vi "Const Lang Default English.vi"() -> (3 "UI Descriptions":T1={"Main Panel"={"Title"={"Frame Num"={"Name"="Frame Num", "Tip"="", "Description"=""}, "Name"={"Name"="Name", "Tip"="", "Description"=""}}, "Frame Basic"={"pic"={"Name"="pic", "Tip"="", "Description"=""}, "state"={"Name"="state", "Tip"="", "Description"=""}, "wait"={"Name"="wait", "Tip"="", "Description"=""}, "next"={"Name"="next", "Tip"="Next frame number", "Description"="Next frame number  \n999: Return to frame number 0  \n1000: Remove object  \n12XX: Invisible, where XX represents the duration  \nA minus sign indicates direction reversal"}, "dvx"={"Name"="dvx", "Tip"="movement speed", "Description"="Forward (positive) and backward (negative) movement speed"}, "dvy"={"Name"="dvy", "Tip"="movement speed", "Description"="Upward (negative) and downward (positive) movement speed"}, "dvz"={"Name"="dvz", "Tip"="movement speed", "Description"="Vertical movement speed, with the direction determined by the ◆ and □ arrow keys"}, "centerx"={"Name"="centerx", "Tip"="X-axis position of the frame center", "Description"="X-axis position of the frame center (shadow), with direction from left to right"}, "centery"={"Name"="centery", "Tip"="Y-axis position of the frame center", "Description"="Y-axis position of the frame center (shadow), with direction from top to bottom"}, "sound"={"Name"="sound", "Tip"="", "Description"=""}}, "Frame Skill"={"mp"={"Name"="mp", "Tip"="HP/MP Consumption", "Description"="HP/MP Consumption  \nOOXXX: OO represents the tens digit of HP consumption, XXX represents MP consumption  \n100: Consumes 100 MP  \n4300: Consumes 40 HP and 300 MP  \n\nWhen entering a frame using hit_XX:  \n  - Positive values indicate consumption  \n  - Negative values indicate recovery  \n\nWhen entering a frame using next:  \n  - Positive values have no effect  \n  - Negative values indicate consumption"}, "hit_a"={"Name"="hit_a", "Tip"="When pressing Attack, jump to the corresponding frame number", "Description"="When pressing Attack, jump to the corresponding frame number"}, "hit_d"={"Name"="hit_d", "Tip"="When pressing Defense, jump to the corresponding frame number", "Description"="When pressing Defense, jump to the corresponding frame number"}, "hit_j"={"Name"="hit_j", "Tip"="When pressing Jump, jump to the corresponding frame number", "Description"="When pressing Jump, jump to the corresponding frame number"}, "hit_Fa"={"Name"="hit_Fa", "Tip"="When pressing Defense △ Attack, jump to the corresponding frame number", "Description"="When pressing Defense △ Attack, jump to the corresponding frame number"}, "hit_Ua"={"Name"="hit_Ua", "Tip"="When pressing Defense ◆ Attack, jump to the corresponding frame number", "Description"="When pressing Defense ◆ Attack, jump to the corresponding frame number"}, "hit_Da"={"Name"="hit_Da", "Tip"="When pressing Defense □ Attack, jump to the corresponding frame number", "Description"="When pressing Defense □ Attack, jump to the corresponding frame number"}, "hit_Fj"={"Name"="hit_Fj", "Tip"="When pressing Defense △ Jump, jump to the corresponding frame number", "Description"="When pressing Defense △ Jump, jump to the corresponding frame number"}, "hit_Uj"={"Name"="hit_Uj", "Tip"="When pressing Defense ◆ Jump, jump to the corresponding frame number", "Description"="When pressing Defense ◆ Jump, jump to the corresponding frame number"}, "hit_Dj"={"Name"="hit_Dj", "Tip"="When pressing Defense □ Jump, jump to the corresponding frame number", "Description"="When pressing Defense □ Jump, jump to the corresponding frame number"}, "hit_ja"={"Name"="hit_ja", "Tip"="When pressing Defense + Jump + Attack, jump to the corresponding frame number", "Description"="When pressing Defense + Jump + Attack, jump to the corresponding frame number"}}, "bp"={"x"={"Name"="x", "Tip"="X-axis position of mouth bleeding", "Description"="X-axis position of mouth bleeding\nBleeding occurs when HP is less than 1/3"}, "y"={"Name"="y", "Tip"="Y-axis position of mouth bleeding", "Description"="Y-axis position of mouth bleeding\nBleeding occurs when HP is less than 1/3"}}, "w"={"kind"={"Name"="kind", "Tip"="Weapon state\n1: Held in hand  \n2: Held in hand  \n3: Dropped", "Description"="Weapon state\n1: Held in hand  \n2: Held in hand  \n3: Dropped"}, "x"={"Name"="x", "Tip"="X-axis position of the weapon", "Description"="X-axis position of the weapon"}, "y"={"Name"="y", "Tip"="Y-axis position of the weapon", "Description"="Y-axis position of the weapon"}, "weaponact"={"Name"="weaponact", "Tip"="Weapon frame number\nIf outside 20~35, the weapon can be hit", "Description"="Weapon frame number\nIf outside 20~35, the weapon can be hit"}, "cover"={"Name"="cover", "Tip"="0: Weapon in front (overlays the character image)  \n1: Weapon behind (character overlays the weapon image)", "Description"="0: Weapon in front (overlays the character image)  \n1: Weapon behind (character overlays the weapon image)"}, "dvx"={"Name"="dvx", "Tip"="movement speed", "Description"="Forward (positive) and backward (negative) movement speed"}, "dvy"={"Name"="dvy", "Tip"="movement speed", "Description"="Upward (negative) and downward (positive) movement speed"}, "dvz"={"Name"="dvz", "Tip"="movement speed", "Description"="Vertical movement speed, with the direction determined by the ◆ and □ arrow keys"}, "attacking"={"Name"="attacking", "Tip"="Attack state", "Description"="Attack state\n0: No attack  \n1: Attack while standing  \n2: Attack while jumping  \n3: Attack while running  \n4: Attack while jumping forward"}}, "b"={"kind"={"Name"="kind", "Tip"="", "Description"=""}, "x"={"Name"="x", "Tip"="X-axis position of the hitbox", "Description"="X-axis position of the hitbox"}, "y"={"Name"="y", "Tip"="Y-axis position of the hitbox", "Description"="Y-axis position of the hitbox"}, "w"={"Name"="w", "Tip"="Width of the hitbox", "Description"="Width of the hitbox"}, "h"={"Name"="h", "Tip"="Height of the hitbox", "Description"="Height of the hitbox"}, "index"={"Name"="<b> index", "Tip"="body section index", "Description"="body section index"}}, "i"={"kind"={"Name"="kind", "Tip"="Injury Effect", "Description"="Injury Effect\n0: Normal attack / effect attack  \n1: Grab a stunned opponent (state 16)  \n2: Pick up a weapon  \n3: Forced grab  \n4: Attack type when thrown by an enemy  \n5: Weapon type  \n6: If an enemy is within this range, jump to a super_punch frame  \n7: Press Attack to pick up a weapon immediately  \n8: Convert injury to healing, jump to dvx frame  \n9: Reduce HP to zero after hitting an enemy  \n10: Henry's \"Death Symphony\" effect  \n11: Henry's \"Death Symphony\" effect  \n14: Block  \n15: Float  \n16: Freeze"}, "x"={"Name"="x", "Tip"="X-axis position of the hitbox", "Description"="X-axis position of the hitbox"}, "y"={"Name"="y", "Tip"="Y-axis position of the hitbox", "Description"="Y-axis position of the hitbox"}, "w"={"Name"="w", "Tip"="Width of the hitbox", "Description"="Width of the hitbox"}, "h"={"Name"="h", "Tip"="Height of the hitbox", "Description"="Height of the hitbox"}, "zwidth"={"Name"="zwidth", "Tip"="Width of the hitbox along the Z-axis", "Description"="Width of the hitbox along the Z-axis"}, "dvx"={"Name"="dvx", "Tip"="movement speed", "Description"="Forward (positive) and backward (negative) movement speed"}, "dvy"={"Name"="dvy", "Tip"="movement speed", "Description"="Upward (negative) and downward (positive) movement speed"}, "dvz"={"Name"="dvz", "Tip"="movement speed", "Description"="Vertical movement speed, with the direction determined by the ◆ and □ arrow keys"}, "fall"={"Name"="fall", "Tip"="Knockdown value", "Description"="Knockdown value\n1: Enemy pauses briefly, but the value does not accumulate toward stun  \n25: Hitting twice will stun the enemy  \n40: First hit makes the enemy step back, second hit knocks them down  \n60: First hit stuns the enemy, second hit knocks them down  \n70: Forced knockdown  \nNegative value: Does not affect the enemy's action, but grants super armor (enemy shows no hurt animation)"}, "arest"={"Name"="arest", "Tip"="Interval for repeatedly attacking a single enemy\nForcibly disables vrest", "Description"="Interval for repeatedly attacking a single enemy\nForcibly disables vrest"}, "vrest"={"Name"="vrest", "Tip"="Interval for repeatedly attacking multiple enemies\nCannot be used simultaneously with arest\nMinimum value is 4", "Description"="Interval for repeatedly attacking multiple enemies\nCannot be used simultaneously with arest\nMinimum value is 4"}, "bdefend"={"Name"="bdefend", "Tip"="Guard break value", "Description"="Guard break value\nAccumulate up to 60 to break a defending enemy  \n60: Directly breaks guard  \n100: Ignores all defense and hits directly. Items are forcibly destroyed"}, "injury"={"Name"="injury", "Tip"="", "Description"=""}, "effect"={"Name"="effect", "Tip"="Attack special effect (only for kind:0)", "Description"="Attack special effect (only for kind:0)\n0: Fist effect  \n1: Bladed weapon effect  \n2: Fire  \n20: Fire, cannot hit ball attacks  \n21: Fire, can reflect ball attacks; when combined with state 18 (fire), it will not hit allies  \n22: Fire; if dvx is positive, attack direction is inward; if dvx is negative, attack direction is outward  \n23: Hit effect; if dvx is positive, attack direction is inward; if dvx is negative, attack direction is outward  \n3: Freeze  \n30: Freeze; cannot hit state 13 characters (frozen characters)  \n4: Only attacks objects of type: 1, 2, 3, 4, 5, 6"}, "catchingact 1"={"Name"="catchingact 1", "Tip"="Only for kind: 1 (grab stunned enemy), kind: 3 (forced grab)\nAfter grabbing an enemy, jumps to the frame number", "Description"="Only for kind: 1 (grab stunned enemy), kind: 3 (forced grab)\nAfter grabbing an enemy, jumps to the frame number"}, "catchingact 2"={"Name"="catchingact 2", "Tip"="Only for kind: 1 (grab stunned enemy), kind: 3 (forced grab)\nAfter grabbing an enemy, jumps to the frame number", "Description"="Only for kind: 1 (grab stunned enemy), kind: 3 (forced grab)\nAfter grabbing an enemy, jumps to the frame number"}, "caughtact 1"={"Name"="caughtact 1", "Tip"="Only for kind: 1 (grab stunned enemy), kind: 3 (forced grab)\nAfter grabbing an enemy, the enemy's frame number jumps to the frame number", "Description"="Only for kind: 1 (grab stunned enemy), kind: 3 (forced grab)\nAfter grabbing an enemy, jumps to the frame number"}, "caughtact 2"={"Name"="caughtact 2", "Tip"="Only for kind: 1 (grab stunned enemy), kind: 3 (forced grab)\nAfter grabbing an enemy, the enemy's frame number jumps to the frame number", "Description"="Only for kind: 1 (grab stunned enemy), kind: 3 (forced grab)\nAfter grabbing an enemy, the enemy's frame number jumps to the frame number"}, "index"={"Name"="<i> index", "Tip"="injury section index", "Description"="injury section index"}}, "o"={"kind"={"Name"="kind", "Tip"="Creation type", "Description"="Creation type\n1: Dropped  \n2: Held in hand"}, "x"={"Name"="x", "Tip"="X-axis position of the object, with direction from left to right", "Description"="X-axis position of the object, with direction from left to right"}, "y"={"Name"="y", "Tip"="Y-axis position of the object, with direction from top to bottom", "Description"="Y-axis position of the object, with direction from top to bottom"}, "action"={"Name"="action", "Tip"="Frame number of the object", "Description"="Frame number of the object"}, "dvx"={"Name"="dvx", "Tip"="movement speed", "Description"="Forward (positive) and backward (negative) movement speed of the object"}, "dvy"={"Name"="dvy", "Tip"="movement speed", "Description"="Upward (negative) and downward (positive) movement speed of the object"}, "dvz"={"Name"="dvz", "Tip"="movement speed", "Description"="Vertical movement speed of the object, with direction determined by the ◆ and □ arrow keys"}, "oid"={"Name"="oid", "Tip"="Object ID", "Description"="Object ID"}, "facing"={"Name"="facing", "Tip"="Object quantity and direction", "Description"="Object quantity and direction\nOOX: OO represents the quantity. X represents the direction, where 0 = forward, 1 = reverse"}}, "c"={"kind"={"Name"="kind", "Tip"="Grab state", "Description"="1: Grabber  \n2: Grabbed"}, "x"={"Name"="x", "Tip"="X-axis position of the grabber/grabbed", "Description"="X-axis position of the grabber/grabbed"}, "y"={"Name"="y", "Tip"="Y-axis position of the grabber/grabbed", "Description"="Y-axis position of the grabber/grabbed"}, "injury"={"Name"="injury", "Tip"="Damage\nPositive value: Causes injury with hit pause effect  \nNegative value: Causes injury without hit pause effect", "Description"="Damage\nPositive value: Causes injury with hit pause effect  \nNegative value: Causes injury without hit pause effect"}, "cover"={"Name"="cover", "Tip"="Layer order\n10: Grabbed character behind  \n11: Grabbed character in front", "Description"="Layer order\n10: Grabbed character behind  \n11: Grabbed character in front"}, "vaction"={"Name"="vaction", "Tip"="Frame number of the grabbed character", "Description"="Frame number of the grabbed character"}, "aaction"={"Name"="aaction", "Tip"="When pressing Attack, jump to the corresponding frame number", "Description"="When pressing Attack, jump to the corresponding frame number"}, "taction"={"Name"="taction", "Tip"="When pressing △ + Attack, jump to the corresponding frame number", "Description"="When pressing △ + Attack, jump to the corresponding frame number"}, "hurtable"={"Name"="hurtable", "Tip"="Whether the grabbed character can be hit by others\n0: No  \n1: Yes", "Description"="Whether the grabbed character can be hit by others\n0: No  \n1: Yes"}, "decrease"={"Name"="decrease", "Tip"="Decrement value for grab duration (negative value), total duration is 301", "Description"="Decrement value for grab duration (negative value), total duration is 301"}, "fronthurtact"={"Name"="fronthurtact", "Tip"="Jump to Frame number after being hit from the front", "Description"="Jump to Frame number after being hit from the front"}, "backhurtact"={"Name"="backhurtact", "Tip"="Jump to Frame number after being hit from the back", "Description"="Jump to Frame number after being hit from the back"}, "throwvx"={"Name"="throwvx", "Tip"="X-direction speed when thrown", "Description"="X-direction speed when thrown"}, "throwvy"={"Name"="throwvy", "Tip"="Y-direction speed when thrown", "Description"="Y-direction speed when thrown"}, "throwvz"={"Name"="throwvz", "Tip"="Z-direction speed when thrown, with direction determined by the ◆ and □ arrow keys", "Description"="Z-direction speed when thrown, with direction determined by the ◆ and □ arrow keys"}, "throwinjury"={"Name"="throwinjury", "Tip"="", "Description"=""}, "dircontrol"={"Name"="dircontrol", "Tip"="", "Description"=""}}, "Other"={"File Path"={"Name"="File Path", "Tip"="", "Description"=""}, "GoTo"={"Name"="Go to Frame", "Tip"="", "Description"=""}, "Apply Change"={"Name"="Apply Change", "Tip"="", "Description"=""}, "To Next Frame"={"Name"="To Next Frame", "Tip"="", "Description"=""}, "Sound Play"={"Name"="Play", "Tip"="", "Description"=""}}, "Menu"={"File"={"Name"="File", "Tip"="", "Description"=""}, "Open File"={"Name"="Open File", "Tip"="", "Description"=""}, "Save File"={"Name"="Save File", "Tip"="", "Description"=""}, "Exit"={"Name"="Exit", "Tip"="", "Description"=""}, "Settings"={"Name"="Settings", "Tip"="", "Description"=""}, "Preferences"={"Name"="Preferences", "Tip"="", "Description"=""}, "Tool"={"Name"="Tool", "Tip"="", "Description"=""}, "PNG Json Generator"={"Name"="PNG Json Generator", "Tip"="", "Description"=""}, "Help"={"Name"="Help", "Tip"="", "Description"=""}, "Show Context Help"={"Name"="Show Context Help", "Tip"="", "Description"=""}}}, "Configuration Window"={"Tab"={"Main Page"={"Name"="Main", "Tip"="", "Description"=""}, "Image Page"={"Name"="Image", "Tip"="", "Description"=""}}, "Main"={"Language"={"Name"="Language", "Tip"="", "Description"=""}, "Save"={"Name"="Save", "Tip"="", "Description"=""}, "Cancel"={"Name"="Cancel", "Tip"="", "Description"=""}}, "Path"={"Reset"={"Name"="Reset to Steam Path", "Tip"="", "Description"=""}, "Path Data"={"Name"="_res_data Folder Path", "Tip"="", "Description"=""}, "Path Png"={"Name"="_res_pngs Folder Path", "Tip"="", "Description"=""}, "Path Mp3"={"Name"="mp3 Folder Path", "Tip"="", "Description"=""}}, "Image"={"Center Point"={"Name"={"Name"="Center Point:", "Tip"="", "Description"=""}, "Size"={"Name"="Size", "Tip"="", "Description"=""}, "Color"={"Name"="Color", "Tip"="", "Description"=""}, "Enable"={"Name"="Enable", "Tip"="", "Description"=""}}, "bp Point"={"Name"={"Name"="<bp> Point:", "Tip"="", "Description"=""}, "Size"={"Name"="Size", "Tip"="", "Description"=""}, "Color"={"Name"="Color", "Tip"="", "Description"=""}, "Enable"={"Name"="Enable", "Tip"="", "Description"=""}}, "w Point"={"Name"={"Name"="<w> Point:", "Tip"="", "Description"=""}, "Size"={"Name"="Size", "Tip"="", "Description"=""}, "Color"={"Name"="Color", "Tip"="", "Description"=""}, "Enable"={"Name"="Enable", "Tip"="", "Description"=""}}, "b Box"={"Name"={"Name"="<b> Box:", "Tip"="", "Description"=""}, "Fill Color"={"Name"="Fill Color", "Tip"="", "Description"=""}, "Border Color"={"Name"="Border Color", "Tip"="", "Description"=""}, "Enable"={"Name"="Enable", "Tip"="", "Description"=""}}, "i Box"={"Name"={"Name"="<i> Box:", "Tip"="", "Description"=""}, "Fill Color"={"Name"="Fill Color", "Tip"="", "Description"=""}, "Border Color"={"Name"="Border Color", "Tip"="", "Description"=""}, "Enable"={"Name"="Enable", "Tip"="", "Description"=""}}, "o Point"={"Name"={"Name"="<o> Point:", "Tip"="", "Description"=""}, "Size"={"Name"="Size", "Tip"="", "Description"=""}, "Color"={"Name"="Color", "Tip"="", "Description"=""}, "Enable"={"Name"="Enable", "Tip"="", "Description"=""}}, "c Point"={"Name"={"Name"="<c> Point:", "Tip"="", "Description"=""}, "Size"={"Name"="Size", "Tip"="", "Description"=""}, "Color"={"Name"="Color", "Tip"="", "Description"=""}, "Enable"={"Name"="Enable", "Tip"="", "Description"=""}}}}})   [LabVIEW 2018, in "Framework.lvlib" / "Framework.lvclass"]
uses:
  Framework.lvclass
  Const Lang Setting.ctl
  Const Lang MainWnd.ctl
  Const Lang MainWnd Frame Title.ctl
  Const Lang Property.ctl
  Const Lang MainWnd Frame Basic.ctl
  Const Lang MainWnd Frame Skill.ctl
  Const Lang MainWnd Frame bp.ctl
  Const Lang MainWnd Frame w.ctl
  Const Lang MainWnd Frame b.ctl
  Const Lang MainWnd Frame i.ctl
  Const Lang MainWnd Frame o.ctl
  Const Lang MainWnd Frame c.ctl
  Const Lang MainWnd Other.ctl
  Const Lang MainWnd Menu.ctl
  Const Lang CfgWnd.ctl
  Const Lang CfgWnd Tab.ctl
  Const Lang CfgWnd Main.ctl
  Const Lang CfgWnd Path.ctl
  Const Lang CfgWnd Image.ctl
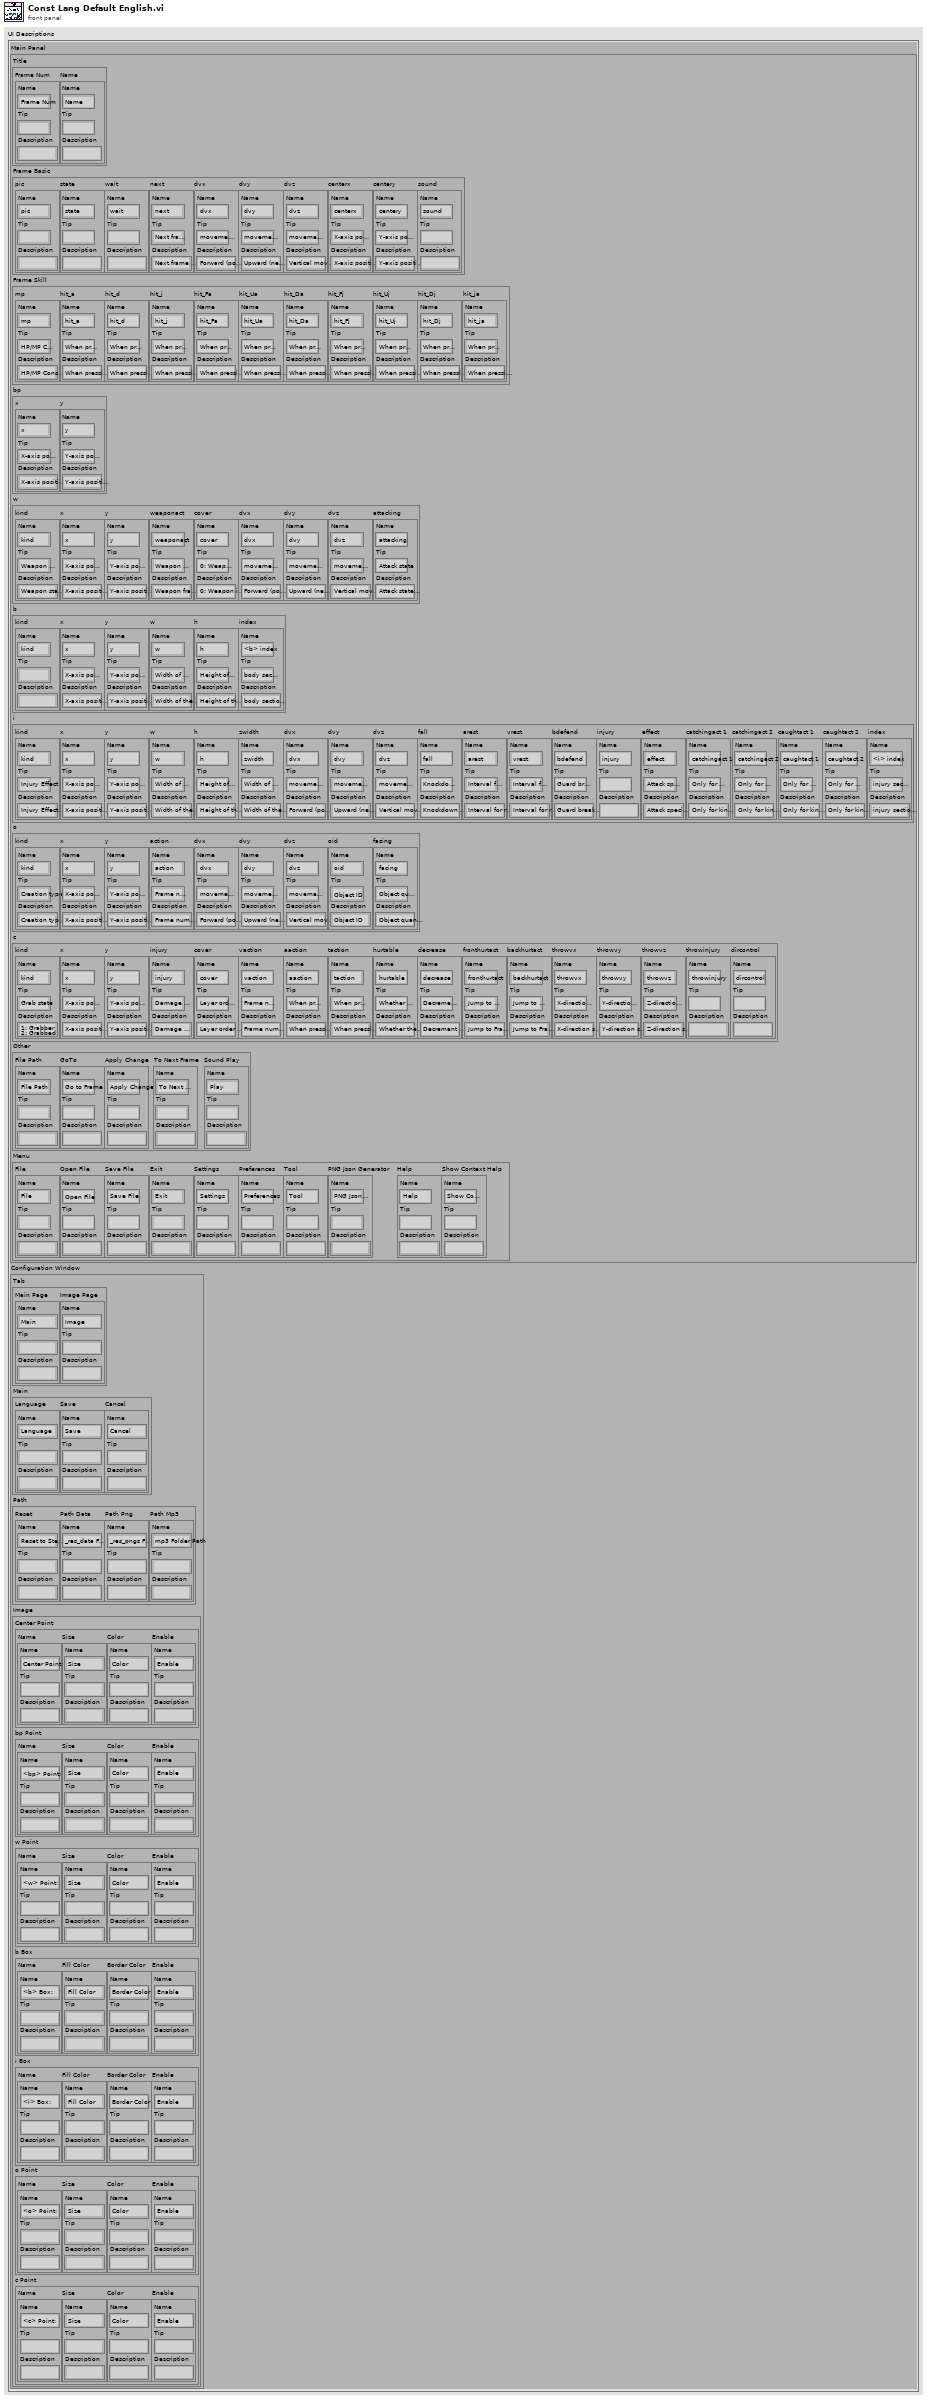
[diagram p1: front panel]
types:
  T1 = typedef "Framework.lvlib/Framework.lvclass/Const Lang Setting.ctl" = cluster{"Main Panel":T2, "Configuration Window":T15}
  T2 = typedef "Framework.lvlib/Framework.lvclass/Const Lang MainWnd.ctl" = cluster{"Title":T3, "Frame Basic":T5, "Frame Skill":T6, "bp":T7, "w":T8, "b":T9, "i":T10, "o":T11, "c":T12, "Other":T13, "Menu":T14}
  T3 = typedef "Framework.lvlib/Framework.lvclass/Const Lang MainWnd Frame Title.ctl" = cluster{"Frame Num":T4, "Name":T4}
  T4 = typedef "Framework.lvlib/Framework.lvclass/Const Lang Property.ctl" = cluster{"Name":string, "Tip":string, "Description":string}
  T5 = typedef "Framework.lvlib/Framework.lvclass/Const Lang MainWnd Frame Basic.ctl" = cluster{"pic":T4, "state":T4, "wait":T4, "next":T4, "dvx":T4, "dvy":T4, "dvz":T4, "centerx":T4, "centery":T4, "sound":T4}
  T6 = typedef "Framework.lvlib/Framework.lvclass/Const Lang MainWnd Frame Skill.ctl" = cluster{"mp":T4, "hit_a":T4, "hit_d":T4, "hit_j":T4, "hit_Fa":T4, "hit_Ua":T4, "hit_Da":T4, "hit_Fj":T4, "hit_Uj":T4, "hit_Dj":T4, "hit_ja":T4}
  T7 = typedef "Framework.lvlib/Framework.lvclass/Const Lang MainWnd Frame bp.ctl" = cluster{"x":T4, "y":T4}
  T8 = typedef "Framework.lvlib/Framework.lvclass/Const Lang MainWnd Frame w.ctl" = cluster{"kind":T4, "x":T4, "y":T4, "weaponact":T4, "cover":T4, "dvx":T4, "dvy":T4, "dvz":T4, "attacking":T4}
  T9 = typedef "Framework.lvlib/Framework.lvclass/Const Lang MainWnd Frame b.ctl" = cluster{"kind":T4, "x":T4, "y":T4, "w":T4, "h":T4, "index":T4}
  T10 = typedef "Framework.lvlib/Framework.lvclass/Const Lang MainWnd Frame i.ctl" = cluster{"kind":T4, "x":T4, "y":T4, "w":T4, "h":T4, "zwidth":T4, "dvx":T4, "dvy":T4, "dvz":T4, "fall":T4, "arest":T4, "vrest":T4, "bdefend":T4, "injury":T4, "effect":T4, "catchingact 1":T4, "catchingact 2":T4, "caughtact 1":T4, "caughtact 2":T4, "index":T4}
  T11 = typedef "Framework.lvlib/Framework.lvclass/Const Lang MainWnd Frame o.ctl" = cluster{"kind":T4, "x":T4, "y":T4, "action":T4, "dvx":T4, "dvy":T4, "dvz":T4, "oid":T4, "facing":T4}
  T12 = typedef "Framework.lvlib/Framework.lvclass/Const Lang MainWnd Frame c.ctl" = cluster{"kind":T4, "x":T4, "y":T4, "injury":T4, "cover":T4, "vaction":T4, "aaction":T4, "taction":T4, "hurtable":T4, "decrease":T4, "fronthurtact":T4, "backhurtact":T4, "throwvx":T4, "throwvy":T4, "throwvz":T4, "throwinjury":T4, "dircontrol":T4}
  T13 = typedef "Framework.lvlib/Framework.lvclass/Const Lang MainWnd Other.ctl" = cluster{"File Path":T4, "GoTo":T4, "Apply Change":T4, "To Next Frame":T4, "Sound Play":T4}
  T14 = typedef "Framework.lvlib/Framework.lvclass/Const Lang MainWnd Menu.ctl" = cluster{"File":T4, "Open File":T4, "Save File":T4, "Exit":T4, "Settings":T4, "Preferences":T4, "Tool":T4, "PNG Json Generator":T4, "Help":T4, "Show Context Help":T4}
  T15 = typedef "Framework.lvlib/Framework.lvclass/Const Lang CfgWnd.ctl" = cluster{"Tab":T16, "Main":T17, "Path":T18, "Image":T19}
  T16 = typedef "Framework.lvlib/Framework.lvclass/Const Lang CfgWnd Tab.ctl" = cluster{"Main Page":T4, "Image Page":T4}
  T17 = typedef "Framework.lvlib/Framework.lvclass/Const Lang CfgWnd Main.ctl" = cluster{"Language":T4, "Save":T4, "Cancel":T4}
  T18 = typedef "Framework.lvlib/Framework.lvclass/Const Lang CfgWnd Path.ctl" = cluster{"Reset":T4, "Path Data":T4, "Path Png":T4, "Path Mp3":T4}
  T19 = typedef "Framework.lvlib/Framework.lvclass/Const Lang CfgWnd Image.ctl" = cluster{"Center Point":cluster{"Name":T4, "Size":T4, "Color":T4, "Enable":T4}, "bp Point":cluster{"Name":T4, "Size":T4, "Color":T4, "Enable":T4}, "w Point":cluster{"Name":T4, "Size":T4, "Color":T4, "Enable":T4}, "b Box":cluster{"Name":T4, "Fill Color":T4, "Border Color":T4, "Enable":T4}, "i Box":cluster{"Name":T4, "Fill Color":T4, "Border Color":T4, "Enable":T4}, "o Point":cluster{"Name":T4, "Size":T4, "Color":T4, "Enable":T4}, "c Point":cluster{"Name":T4, "Size":T4, "Color":T4, "Enable":T4}}
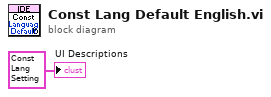
[diagram p0: block diagram]
diagram:
  "UI Descriptions" <- T1 {"Main Panel"={"Title"={"Frame Num"={"Name"="Frame Num", "Tip"="", "Description"=""}, "Name"={"Name"="Name", "Tip"="", "Description"=""}}, "Frame Basic"={"pic"={"Name"="pic", "Tip"="", "Description"=""}, "state"={"Name"="state", "Tip"="", "Description"=""}, "wait"={"Name"="wait", "Tip"="", "Description"=""}, "next"={"Name"="next", "Tip"="Next frame number", "Description"="Next frame number  \n999: Return to frame number 0  \n1000: Remove object  \n12XX: Invisible, where XX represents the duration  \nA minus sign indicates direction reversal"}, "dvx"={"Name"="dvx", "Tip"="movement speed", "Description"="Forward (positive) and backward (negative) movement speed"}, "dvy"={"Name"="dvy", "Tip"="movement speed", "Description"="Upward (negative) and downward (positive) movement speed"}, "dvz"={"Name"="dvz", "Tip"="movement speed", "Description"="Vertical movement speed, with the direction determined by the ◆ and □ arrow keys"}, "centerx"={"Name"="centerx", "Tip"="X-axis position of the frame center", "Description"="X-axis position of the frame center (shadow), with direction from left to right"}, "centery"={"Name"="centery", "Tip"="Y-axis position of the frame center", "Description"="Y-axis position of the frame center (shadow), with direction from top to bottom"}, "sound"={"Name"="sound", "Tip"="", "Description"=""}}, "Frame Skill"={"mp"={"Name"="mp", "Tip"="HP/MP Consumption", "Description"="HP/MP Consumption  \nOOXXX: OO represents the tens digit of HP consumption, XXX represents MP consumption  \n100: Consumes 100 MP  \n4300: Consumes 40 HP and 300 MP  \n\nWhen entering a frame using hit_XX:  \n  - Positive values indicate consumption  \n  - Negative values indicate recovery  \n\nWhen entering a frame using next:  \n  - Positive values have no effect  \n  - Negative values indicate consumption"}, "hit_a"={"Name"="hit_a", "Tip"="When pressing Attack, jump to the corresponding frame number", "Description"="When pressing Attack, jump to the corresponding frame number"}, "hit_d"={"Name"="hit_d", "Tip"="When pressing Defense, jump to the corresponding frame number", "Description"="When pressing Defense, jump to the corresponding frame number"}, "hit_j"={"Name"="hit_j", "Tip"="When pressing Jump, jump to the corresponding frame number", "Description"="When pressing Jump, jump to the corresponding frame number"}, "hit_Fa"={"Name"="hit_Fa", "Tip"="When pressing Defense △ Attack, jump to the corresponding frame number", "Description"="When pressing Defense △ Attack, jump to the corresponding frame number"}, "hit_Ua"={"Name"="hit_Ua", "Tip"="When pressing Defense ◆ Attack, jump to the corresponding frame number", "Description"="When pressing Defense ◆ Attack, jump to the corresponding frame number"}, "hit_Da"={"Name"="hit_Da", "Tip"="When pressing Defense □ Attack, jump to the corresponding frame number", "Description"="When pressing Defense □ Attack, jump to the corresponding frame number"}, "hit_Fj"={"Name"="hit_Fj", "Tip"="When pressing Defense △ Jump, jump to the corresponding frame number", "Description"="When pressing Defense △ Jump, jump to the corresponding frame number"}, "hit_Uj"={"Name"="hit_Uj", "Tip"="When pressing Defense ◆ Jump, jump to the corresponding frame number", "Description"="When pressing Defense ◆ Jump, jump to the corresponding frame number"}, "hit_Dj"={"Name"="hit_Dj", "Tip"="When pressing Defense □ Jump, jump to the corresponding frame number", "Description"="When pressing Defense □ Jump, jump to the corresponding frame number"}, "hit_ja"={"Name"="hit_ja", "Tip"="When pressing Defense + Jump + Attack, jump to the corresponding frame number", "Description"="When pressing Defense + Jump + Attack, jump to the corresponding frame number"}}, "bp"={"x"={"Name"="x", "Tip"="X-axis position of mouth bleeding", "Description"="X-axis position of mouth bleeding\nBleeding occurs when HP is less than 1/3"}, "y"={"Name"="y", "Tip"="Y-axis position of mouth bleeding", "Description"="Y-axis position of mouth bleeding\nBleeding occurs when HP is less than 1/3"}}, "w"={"kind"={"Name"="kind", "Tip"="Weapon state\n1: Held in hand  \n2: Held in hand  \n3: Dropped", "Description"="Weapon state\n1: Held in hand  \n2: Held in hand  \n3: Dropped"}, "x"={"Name"="x", "Tip"="X-axis position of the weapon", "Description"="X-axis position of the weapon"}, "y"={"Name"="y", "Tip"="Y-axis position of the weapon", "Description"="Y-axis position of the weapon"}, "weaponact"={"Name"="weaponact", "Tip"="Weapon frame number\nIf outside 20~35, the weapon can be hit", "Description"="Weapon frame number\nIf outside 20~35, the weapon can be hit"}, "cover"={"Name"="cover", "Tip"="0: Weapon in front (overlays the character image)  \n1: Weapon behind (character overlays the weapon image)", "Description"="0: Weapon in front (overlays the character image)  \n1: Weapon behind (character overlays the weapon image)"}, "dvx"={"Name"="dvx", "Tip"="movement speed", "Description"="Forward (positive) and backward (negative) movement speed"}, "dvy"={"Name"="dvy", "Tip"="movement speed", "Description"="Upward (negative) and downward (positive) movement speed"}, "dvz"={"Name"="dvz", "Tip"="movement speed", "Description"="Vertical movement speed, with the direction determined by the ◆ and □ arrow keys"}, "attacking"={"Name"="attacking", "Tip"="Attack state", "Description"="Attack state\n0: No attack  \n1: Attack while standing  \n2: Attack while jumping  \n3: Attack while running  \n4: Attack while jumping forward"}}, "b"={"kind"={"Name"="kind", "Tip"="", "Description"=""}, "x"={"Name"="x", "Tip"="X-axis position of the hitbox", "Description"="X-axis position of the hitbox"}, "y"={"Name"="y", "Tip"="Y-axis position of the hitbox", "Description"="Y-axis position of the hitbox"}, "w"={"Name"="w", "Tip"="Width of the hitbox", "Description"="Width of the hitbox"}, "h"={"Name"="h", "Tip"="Height of the hitbox", "Description"="Height of the hitbox"}, "index"={"Name"="<b> index", "Tip"="body section index", "Description"="body section index"}}, "i"={"kind"={"Name"="kind", "Tip"="Injury Effect", "Description"="Injury Effect\n0: Normal attack / effect attack  \n1: Grab a stunned opponent (state 16)  \n2: Pick up a weapon  \n3: Forced grab  \n4: Attack type when thrown by an enemy  \n5: Weapon type  \n6: If an enemy is within this range, jump to a super_punch frame  \n7: Press Attack to pick up a weapon immediately  \n8: Convert injury to healing, jump to dvx frame  \n9: Reduce HP to zero after hitting an enemy  \n10: Henry's \"Death Symphony\" effect  \n11: Henry's \"Death Symphony\" effect  \n14: Block  \n15: Float  \n16: Freeze"}, "x"={"Name"="x", "Tip"="X-axis position of the hitbox", "Description"="X-axis position of the hitbox"}, "y"={"Name"="y", "Tip"="Y-axis position of the hitbox", "Description"="Y-axis position of the hitbox"}, "w"={"Name"="w", "Tip"="Width of the hitbox", "Description"="Width of the hitbox"}, "h"={"Name"="h", "Tip"="Height of the hitbox", "Description"="Height of the hitbox"}, "zwidth"={"Name"="zwidth", "Tip"="Width of the hitbox along the Z-axis", "Description"="Width of the hitbox along the Z-axis"}, "dvx"={"Name"="dvx", "Tip"="movement speed", "Description"="Forward (positive) and backward (negative) movement speed"}, "dvy"={"Name"="dvy", "Tip"="movement speed", "Description"="Upward (negative) and downward (positive) movement speed"}, "dvz"={"Name"="dvz", "Tip"="movement speed", "Description"="Vertical movement speed, with the direction determined by the ◆ and □ arrow keys"}, "fall"={"Name"="fall", "Tip"="Knockdown value", "Description"="Knockdown value\n1: Enemy pauses briefly, but the value does not accumulate toward stun  \n25: Hitting twice will stun the enemy  \n40: First hit makes the enemy step back, second hit knocks them down  \n60: First hit stuns the enemy, second hit knocks them down  \n70: Forced knockdown  \nNegative value: Does not affect the enemy's action, but grants super armor (enemy shows no hurt animation)"}, "arest"={"Name"="arest", "Tip"="Interval for repeatedly attacking a single enemy\nForcibly disables vrest", "Description"="Interval for repeatedly attacking a single enemy\nForcibly disables vrest"}, "vrest"={"Name"="vrest", "Tip"="Interval for repeatedly attacking multiple enemies\nCannot be used simultaneously with arest\nMinimum value is 4", "Description"="Interval for repeatedly attacking multiple enemies\nCannot be used simultaneously with arest\nMinimum value is 4"}, "bdefend"={"Name"="bdefend", "Tip"="Guard break value", "Description"="Guard break value\nAccumulate up to 60 to break a defending enemy  \n60: Directly breaks guard  \n100: Ignores all defense and hits directly. Items are forcibly destroyed"}, "injury"={"Name"="injury", "Tip"="", "Description"=""}, "effect"={"Name"="effect", "Tip"="Attack special effect (only for kind:0)", "Description"="Attack special effect (only for kind:0)\n0: Fist effect  \n1: Bladed weapon effect  \n2: Fire  \n20: Fire, cannot hit ball attacks  \n21: Fire, can reflect ball attacks; when combined with state 18 (fire), it will not hit allies  \n22: Fire; if dvx is positive, attack direction is inward; if dvx is negative, attack direction is outward  \n23: Hit effect; if dvx is positive, attack direction is inward; if dvx is negative, attack direction is outward  \n3: Freeze  \n30: Freeze; cannot hit state 13 characters (frozen characters)  \n4: Only attacks objects of type: 1, 2, 3, 4, 5, 6"}, "catchingact 1"={"Name"="catchingact 1", "Tip"="Only for kind: 1 (grab stunned enemy), kind: 3 (forced grab)\nAfter grabbing an enemy, jumps to the frame number", "Description"="Only for kind: 1 (grab stunned enemy), kind: 3 (forced grab)\nAfter grabbing an enemy, jumps to the frame number"}, "catchingact 2"={"Name"="catchingact 2", "Tip"="Only for kind: 1 (grab stunned enemy), kind: 3 (forced grab)\nAfter grabbing an enemy, jumps to the frame number", "Description"="Only for kind: 1 (grab stunned enemy), kind: 3 (forced grab)\nAfter grabbing an enemy, jumps to the frame number"}, "caughtact 1"={"Name"="caughtact 1", "Tip"="Only for kind: 1 (grab stunned enemy), kind: 3 (forced grab)\nAfter grabbing an enemy, the enemy's frame number jumps to the frame number", "Description"="Only for kind: 1 (grab stunned enemy), kind: 3 (forced grab)\nAfter grabbing an enemy, jumps to the frame number"}, "caughtact 2"={"Name"="caughtact 2", "Tip"="Only for kind: 1 (grab stunned enemy), kind: 3 (forced grab)\nAfter grabbing an enemy, the enemy's frame number jumps to the frame number", "Description"="Only for kind: 1 (grab stunned enemy), kind: 3 (forced grab)\nAfter grabbing an enemy, the enemy's frame number jumps to the frame number"}, "index"={"Name"="<i> index", "Tip"="injury section index", "Description"="injury section index"}}, "o"={"kind"={"Name"="kind", "Tip"="Creation type", "Description"="Creation type\n1: Dropped  \n2: Held in hand"}, "x"={"Name"="x", "Tip"="X-axis position of the object, with direction from left to right", "Description"="X-axis position of the object, with direction from left to right"}, "y"={"Name"="y", "Tip"="Y-axis position of the object, with direction from top to bottom", "Description"="Y-axis position of the object, with direction from top to bottom"}, "action"={"Name"="action", "Tip"="Frame number of the object", "Description"="Frame number of the object"}, "dvx"={"Name"="dvx", "Tip"="movement speed", "Description"="Forward (positive) and backward (negative) movement speed of the object"}, "dvy"={"Name"="dvy", "Tip"="movement speed", "Description"="Upward (negative) and downward (positive) movement speed of the object"}, "dvz"={"Name"="dvz", "Tip"="movement speed", "Description"="Vertical movement speed of the object, with direction determined by the ◆ and □ arrow keys"}, "oid"={"Name"="oid", "Tip"="Object ID", "Description"="Object ID"}, "facing"={"Name"="facing", "Tip"="Object quantity and direction", "Description"="Object quantity and direction\nOOX: OO represents the quantity. X represents the direction, where 0 = forward, 1 = reverse"}}, "c"={"kind"={"Name"="kind", "Tip"="Grab state", "Description"="1: Grabber  \n2: Grabbed"}, "x"={"Name"="x", "Tip"="X-axis position of the grabber/grabbed", "Description"="X-axis position of the grabber/grabbed"}, "y"={"Name"="y", "Tip"="Y-axis position of the grabber/grabbed", "Description"="Y-axis position of the grabber/grabbed"}, "injury"={"Name"="injury", "Tip"="Damage\nPositive value: Causes injury with hit pause effect  \nNegative value: Causes injury without hit pause effect", "Description"="Damage\nPositive value: Causes injury with hit pause effect  \nNegative value: Causes injury without hit pause effect"}, "cover"={"Name"="cover", "Tip"="Layer order\n10: Grabbed character behind  \n11: Grabbed character in front", "Description"="Layer order\n10: Grabbed character behind  \n11: Grabbed character in front"}, "vaction"={"Name"="vaction", "Tip"="Frame number of the grabbed character", "Description"="Frame number of the grabbed character"}, "aaction"={"Name"="aaction", "Tip"="When pressing Attack, jump to the corresponding frame number", "Description"="When pressing Attack, jump to the corresponding frame number"}, "taction"={"Name"="taction", "Tip"="When pressing △ + Attack, jump to the corresponding frame number", "Description"="When pressing △ + Attack, jump to the corresponding frame number"}, "hurtable"={"Name"="hurtable", "Tip"="Whether the grabbed character can be hit by others\n0: No  \n1: Yes", "Description"="Whether the grabbed character can be hit by others\n0: No  \n1: Yes"}, "decrease"={"Name"="decrease", "Tip"="Decrement value for grab duration (negative value), total duration is 301", "Description"="Decrement value for grab duration (negative value), total duration is 301"}, "fronthurtact"={"Name"="fronthurtact", "Tip"="Jump to Frame number after being hit from the front", "Description"="Jump to Frame number after being hit from the front"}, "backhurtact"={"Name"="backhurtact", "Tip"="Jump to Frame number after being hit from the back", "Description"="Jump to Frame number after being hit from the back"}, "throwvx"={"Name"="throwvx", "Tip"="X-direction speed when thrown", "Description"="X-direction speed when thrown"}, "throwvy"={"Name"="throwvy", "Tip"="Y-direction speed when thrown", "Description"="Y-direction speed when thrown"}, "throwvz"={"Name"="throwvz", "Tip"="Z-direction speed when thrown, with direction determined by the ◆ and □ arrow keys", "Description"="Z-direction speed when thrown, with direction determined by the ◆ and □ arrow keys"}, "throwinjury"={"Name"="throwinjury", "Tip"="", "Description"=""}, "dircontrol"={"Name"="dircontrol", "Tip"="", "Description"=""}}, "Other"={"File Path"={"Name"="File Path", "Tip"="", "Description"=""}, "GoTo"={"Name"="Go to Frame", "Tip"="", "Description"=""}, "Apply Change"={"Name"="Apply Change", "Tip"="", "Description"=""}, "To Next Frame"={"Name"="To Next Frame", "Tip"="", "Description"=""}, "Sound Play"={"Name"="Play", "Tip"="", "Description"=""}}, "Menu"={"File"={"Name"="File", "Tip"="", "Description"=""}, "Open File"={"Name"="Open File", "Tip"="", "Description"=""}, "Save File"={"Name"="Save File", "Tip"="", "Description"=""}, "Exit"={"Name"="Exit", "Tip"="", "Description"=""}, "Settings"={"Name"="Settings", "Tip"="", "Description"=""}, "Preferences"={"Name"="Preferences", "Tip"="", "Description"=""}, "Tool"={"Name"="Tool", "Tip"="", "Description"=""}, "PNG Json Generator"={"Name"="PNG Json Generator", "Tip"="", "Description"=""}, "Help"={"Name"="Help", "Tip"="", "Description"=""}, "Show Context Help"={"Name"="Show Context Help", "Tip"="", "Description"=""}}}, "Configuration Window"={"Tab"={"Main Page"={"Name"="Main", "Tip"="", "Description"=""}, "Image Page"={"Name"="Image", "Tip"="", "Description"=""}}, "Main"={"Language"={"Name"="Language", "Tip"="", "Description"=""}, "Save"={"Name"="Save", "Tip"="", "Description"=""}, "Cancel"={"Name"="Cancel", "Tip"="", "Description"=""}}, "Path"={"Reset"={"Name"="Reset to Steam Path", "Tip"="", "Description"=""}, "Path Data"={"Name"="_res_data Folder Path", "Tip"="", "Description"=""}, "Path Png"={"Name"="_res_pngs Folder Path", "Tip"="", "Description"=""}, "Path Mp3"={"Name"="mp3 Folder Path", "Tip"="", "Description"=""}}, "Image"={"Center Point"={"Name"={"Name"="Center Point:", "Tip"="", "Description"=""}, "Size"={"Name"="Size", "Tip"="", "Description"=""}, "Color"={"Name"="Color", "Tip"="", "Description"=""}, "Enable"={"Name"="Enable", "Tip"="", "Description"=""}}, "bp Point"={"Name"={"Name"="<bp> Point:", "Tip"="", "Description"=""}, "Size"={"Name"="Size", "Tip"="", "Description"=""}, "Color"={"Name"="Color", "Tip"="", "Description"=""}, "Enable"={"Name"="Enable", "Tip"="", "Description"=""}}, "w Point"={"Name"={"Name"="<w> Point:", "Tip"="", "Description"=""}, "Size"={"Name"="Size", "Tip"="", "Description"=""}, "Color"={"Name"="Color", "Tip"="", "Description"=""}, "Enable"={"Name"="Enable", "Tip"="", "Description"=""}}, "b Box"={"Name"={"Name"="<b> Box:", "Tip"="", "Description"=""}, "Fill Color"={"Name"="Fill Color", "Tip"="", "Description"=""}, "Border Color"={"Name"="Border Color", "Tip"="", "Description"=""}, "Enable"={"Name"="Enable", "Tip"="", "Description"=""}}, "i Box"={"Name"={"Name"="<i> Box:", "Tip"="", "Description"=""}, "Fill Color"={"Name"="Fill Color", "Tip"="", "Description"=""}, "Border Color"={"Name"="Border Color", "Tip"="", "Description"=""}, "Enable"={"Name"="Enable", "Tip"="", "Description"=""}}, "o Point"={"Name"={"Name"="<o> Point:", "Tip"="", "Description"=""}, "Size"={"Name"="Size", "Tip"="", "Description"=""}, "Color"={"Name"="Color", "Tip"="", "Description"=""}, "Enable"={"Name"="Enable", "Tip"="", "Description"=""}}, "c Point"={"Name"={"Name"="<c> Point:", "Tip"="", "Description"=""}, "Size"={"Name"="Size", "Tip"="", "Description"=""}, "Color"={"Name"="Color", "Tip"="", "Description"=""}, "Enable"={"Name"="Enable", "Tip"="", "Description"=""}}}}} ("UI Descriptions")
